vi "Plot Update.vi"(6 "BluePlotHandle":refnum<class "RocketPlotHandle.lvclass">, 7 "update plot":T2, 8 "error in (no error)":errorcluster, 9 "top array":T5[](array[typedef]), 10 "Oldest Time to Plot (autoscaled)":u64, 11 "refs":T6) -> (0 "error out":errorcluster, 1 "Numerics":dbl[](array[numeric]), 3 "Plot":cluster{dbl[], "Data":dbl[]}[](graph), 5 "RightClickCache.slice":T1[](array[typedef]))   [LabVIEW 2021, in "RocketPlot.lvlib"]
uses:
  RocketPlot.lvlib
  TypeDefs/Plot UI references.ctl
  Classes/RocketPlotHandle/RocketPlotHandle.lvclass
  <userlib>/bjustice/TipStripOOPanel/Classes/TipPanelHandle/TipPanelHandle.lvclass
  TypeDefs/Plot top row.ctl
  TypeDefs/update plot queue data.ctl
  TypeDefs/RightClickType.ctl
  <vilib>/Utility/miscctls.llb/LVPoint32TypeDef.ctl
  TypeDefs/Slice average.ctl
  3bb0a56c-05e9-4756-838c-835a6169e05e.vi
  b137599e-1cd7-4d16-b104-70f5027a024b.vi
  2f37a579-6204-438e-8027-9b28c4813891.vi
  f25a2b61-2115-47b2-97b2-7a0bdbaa418c.vi
  <userlib>/bjustice/Ring Buffer for Time Series Data Strict Accessor/Unix time epoch/Unix_Epoch_in_Labview.vi
  Plot get newest and latest timestamp.vi
  Plot create flatline.vi
  plot Unix to LV epoch.vi
  Decimate data.vi
  Slice Average calc wrapper.vi
  plot Unix to LV epoch.vi/3a8248cf-bec7-4c8d-a232-b35239452a92.vi
  plot Unix to LV epoch.vi/6d88088e-0f8c-482f-b724-f15eac533201.vi
  Decimate calc factors.vi
  Decimate data.vi/10c546bb-84c8-4f1e-93dc-e9aef4c9908a.vi
  Slice Average calc.vi
  Slice Average calc wrapper.vi/b0f39d84-27d9-4b84-b8c3-cf78f35fa78a.vi
  Slice Average calc wrapper.vi/b8f4d68e-665a-4d51-938f-4be5908799fb.vi
  Slice Average calc wrapper.vi/0a7e6c96-3213-4357-8ae2-7647ccf6d38e.vi
  Slice Average calc wrapper.vi/de1cbfd4-f4b0-4655-8da2-e779fdd6673d.vi
  <userlib>/bjustice/Ring Buffer for Time Series Data Strict Accessor/SubVIs/Search for time to keep.vi
  Slice Average calc.vi/aeb3b9b0-3d0b-48fb-8ca9-3c9e8c208765.vi
  Slice Average calc.vi/43998882-4a9d-44ca-a800-b6f182c48d79.vi
  <userlib>/bjustice/Ring Buffer for Time Series Data Strict Accessor/SubVIs/Search for oldest time to keep.vi
  <userlib>/bjustice/Ring Buffer for Time Series Data Strict Accessor/SubVIs/Search for newest time to keep.vi
  <vilib>/Analysis/baseanly.llb/Std Deviation and Variance.vi
  <vilib>/Analysis/8numeric.llb/Uneven Numeric Integration.vi
  nontime x-axis data.vi
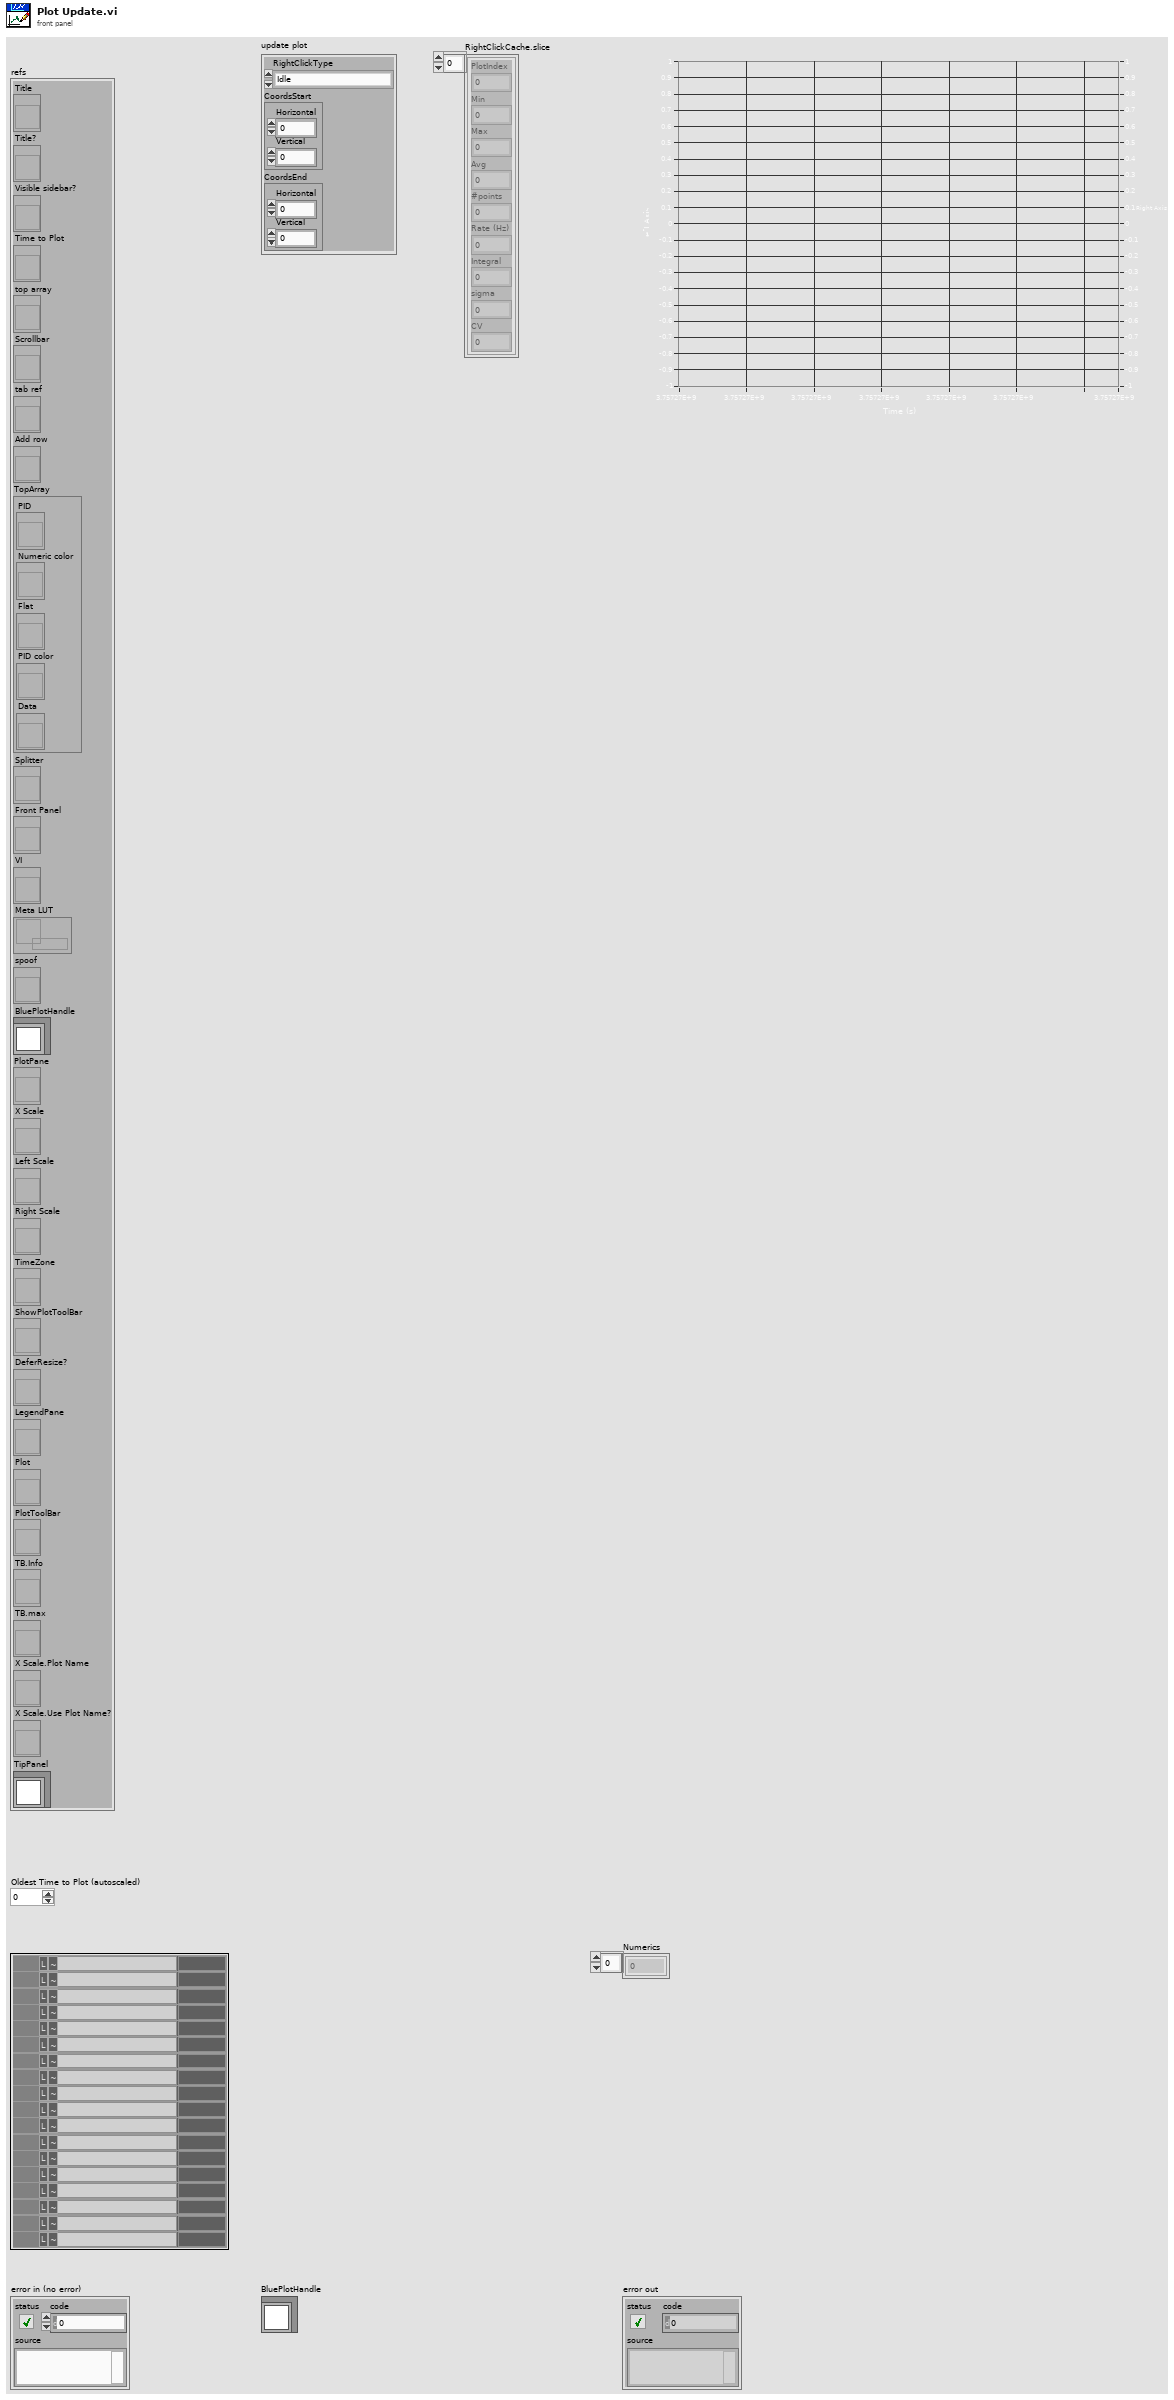
[diagram p1: front panel]
types:
  T1 = typedef "RocketPlot.lvlib/Slice average.ctl" = cluster{"PlotIndex":i32, "Min":dbl, "Max":dbl, "Avg":dbl, "#points":u32, "Rate (Hz)":dbl, "Integral":dbl, "sigma":dbl, "CV":dbl}
  T2 = typedef "RocketPlot.lvlib/update plot queue data.ctl" = cluster{"RightClickType":T3, "CoordsStart":T4, "CoordsEnd":T4}
  T3 = typedef "RocketPlot.lvlib/RightClickType.ctl" = enum16{"Idle", "Delta", "SliceAvg", "Identify"}
  T4 = typedef "LVPoint32TypeDef.ctl" = cluster{"Horizontal":i32, "Vertical":i32}
  T5 = typedef "RocketPlot.lvlib/Plot top row.ctl" = cluster{"PID":string, "index":i32, "PID color":u32, "right axis?":bool, "Flatline?":bool, "Numeric color":u32, "Data":string, "Flat":string}
  T6 = typedef "RocketPlot.lvlib/Plot UI references.ctl" = cluster{"Title":refnum<vi>, "Title?":refnum<vi>, "Visible sidebar?":refnum<vi>, "Time to Plot":refnum<vi>, "top array":refnum<vi>, "Scrollbar":refnum<vi>, "tab ref":refnum<vi>, "Add row":refnum<vi>, "TopArray":cluster{"PID":refnum<vi>, "Numeric color":refnum<vi>, "Flat":refnum<vi>, "PID color":refnum<vi>, "Data":refnum<vi>}, "Splitter":refnum<vi>, "Front Panel":refnum<vi>, "VI":refnum<vi>, "Meta LUT":refnum<data-value>, "spoof":refnum<vi>, "BluePlotHandle":refnum<class "RocketPlotHandle.lvclass">, "PlotPane":refnum<vi>, "X Scale":refnum<vi>, "Left Scale":refnum<vi>, "Right Scale":refnum<vi>, "TimeZone":refnum<vi>, "ShowPlotToolBar":refnum<vi>, "DeferResize?":refnum<vi>, "LegendPane":refnum<vi>, "Plot":refnum<vi>, "PlotToolBar":refnum<vi>, "TB.Info":refnum<vi>, "TB.max":refnum<vi>, "X Scale.Plot Name":refnum<vi>, "X Scale.Use Plot Name?":refnum<vi>, "TipPanel":refnum<class "TipPanelHandle.lvclass">}
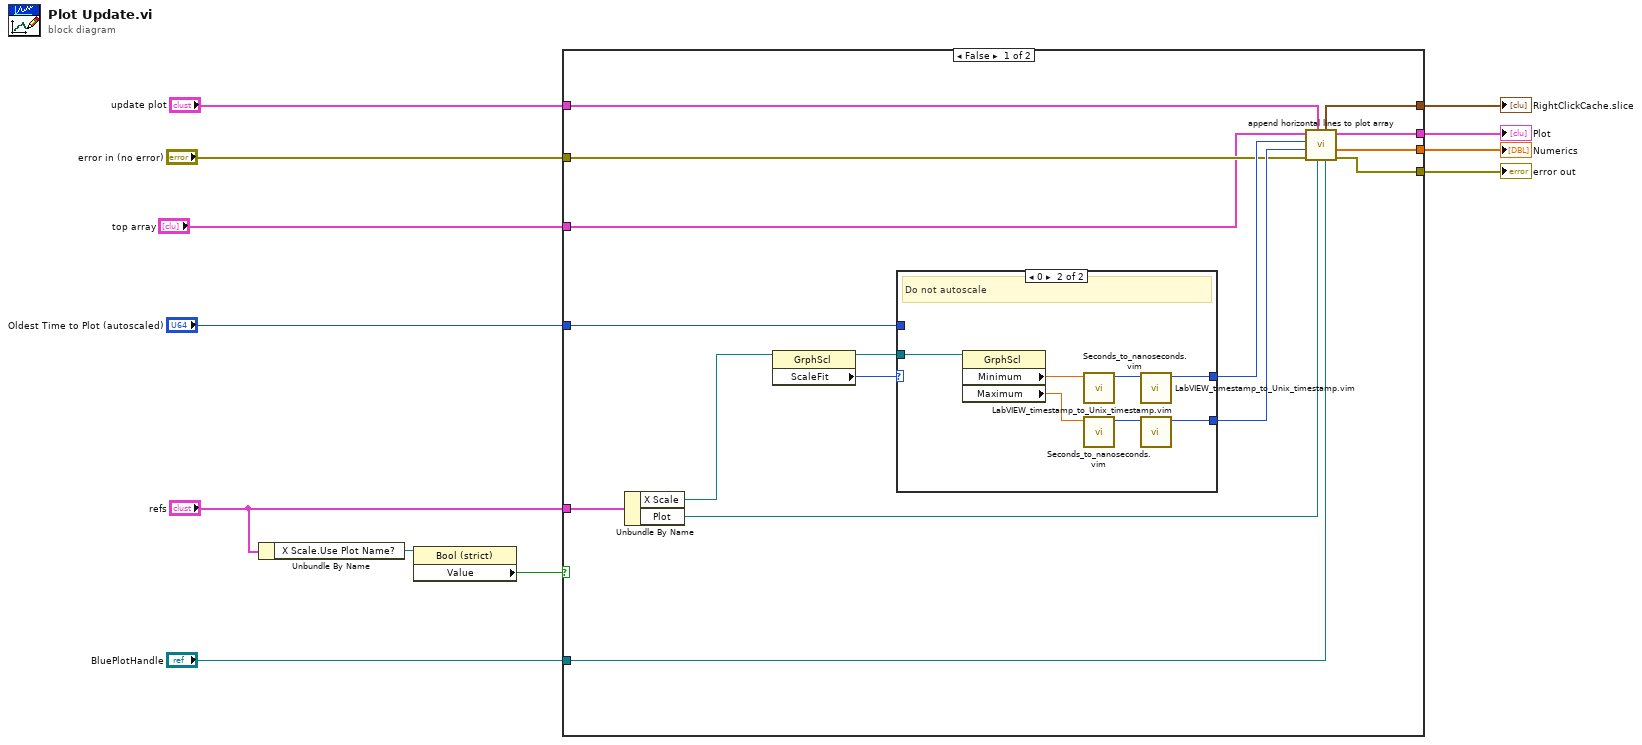
[diagram p0: block diagram]
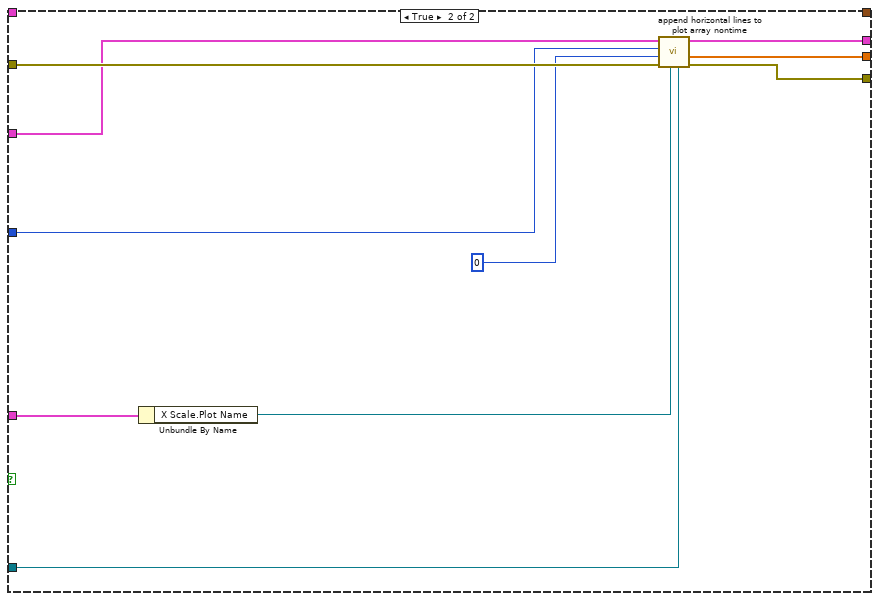
[diagram p3: hidden frame]
diagram:
  n1 = Unbundle By Name("refs") -> ("X Scale.Use Plot Name?"=w4:refnum<vi>)
  n2 = property class="Bool (strict)"(reference=w4) -> ("Value"=w3:bool)  [unwired: 1 in, 2 out]
  n3 = case shown="False" w3 {
    tunnel: [w28 w43] -> w12
    tunnel: [w27 w44] -> w11
    tunnel: "Oldest Time to Plot (autoscaled)" -> [w25 w38]
    tunnel: "error in (no error)" -> [w20 w46]
    tunnel: [w19 w45] -> w8
    tunnel: "top array" -> [w18 w42]
    tunnel: "BluePlotHandle" -> [w17 w40]
    tunnel: "update plot" -> [w15 _]
    tunnel: [w14 _] -> w2
    tunnel: "refs" -> [w13 w41]
    frame False {
      n4 = Unbundle By Name(w13) -> ("X Scale"=w23:refnum<vi>, "Plot"=w16:refnum<vi>)
      n5 = property class="GrphScl"(reference=w23) -> (reference out=w26:refnum<vi>, "ScaleFit"=w24:u8)  [unwired: 1 in, 1 out]
      n6 = case shown="0" w24 {
        tunnel: w26 -> [_ w36]
        tunnel: w25 -> [w29 _]
        tunnel: [w29 w33] -> w22
        tunnel: [_ w30] -> w21
        frame 2, Default {
          # "autoscale"
        }
        frame 0 {
          # "Do not autoscale"
          n7 = property class="GrphScl"(reference=w36) -> ("Minimum"=w34:dbl, "Maximum"=w31:dbl)  [unwired: 1 in, 2 out]
          n8 = call "Seconds_to_nanoseconds.vim"("timestamp (seconds)"=w34) -> ("timestamp (nanoseconds)"=w35:u64)  [unwired: 10 in]
          n9 = call "Seconds_to_nanoseconds.vim"("timestamp (seconds)"=w31) -> ("timestamp (nanoseconds)"=w32:u64)  [unwired: 10 in]
          n10 = call "LabVIEW_timestamp_to_Unix_timestamp.vim"("LabVIEW timestamp (nanoseconds)"=w35) -> ("Unix timestamp (nanoseconds)"=w33:u64)  [unwired: 10 in]
          n11 = call "LabVIEW_timestamp_to_Unix_timestamp.vim"("LabVIEW timestamp (nanoseconds)"=w32) -> ("Unix timestamp (nanoseconds)"=w30:u64)  [unwired: 10 in]
        }
      }
      n12 = call "append horizontal lines to plot array.vi"("BluePlotHandle"=w17, "Plot ref"=w16, "update plot"=w15, "error in (no error)"=w20, "Newest Time to Plot (unix,ns)"=w21, "Oldest Time to Plot (unix,ns)"=w22, "top array"=w18) -> ("error out"=w19:errorcluster, "Numerics"=w28:dbl[], "Plot (LV epoch)"=w27:cluster{dbl[], "Data":dbl[]}[], "RightClickCache.slice"=w14:T1[])  [unwired: 1 in]
    }
    frame True {
      n13 = Unbundle By Name(w41) -> ("X Scale.Plot Name"=w37:refnum<vi>)
      n14 = call "append horizontal lines to plot array nontime.vi"("BluePlotHandle"=w40, "x-axis name"=w37, "error in (no error)"=w46, "Newest Time to Plot (unix,ns)"=u64 0, "Oldest Time to Plot (unix,ns)"=w38, "top array"=w42) -> ("error out"=w45:errorcluster, "Numerics"=w43:dbl[], "Plot (LV epoch)"=w44:cluster{dbl[], "Data":dbl[]}[])  [unwired: 3 in]
    }
  }
  "Numerics" <- w12
  "Plot" <- w11
  "error out" <- w8
  "RightClickCache.slice" <- w2
